vi "Test_WriteValue_InvalidRefnum_Error.vi"(8 "error in (no error)":errorcluster, 11 "TestCase in":refnum<class "TestStreamToDiskTransport.lvclass">) -> (0 "error out":errorcluster, 3 "TestCase out":refnum<class "TestStreamToDiskTransport.lvclass">)   [LabVIEW 2017, in "TestStreamToDiskTransport.lvclass"]
uses:
  TestStreamToDiskTransport.lvclass
  TestStreamToDiskTransport.lvclass/TestStreamToDiskTransport.ctl
  Source/Concrete/StreamToDiskTransport/StreamToDiskTransport.lvclass/StreamToDiskTransport.ctl
  <vilib>/Utility/error.llb/Clear Errors.vi
  Source/Concrete/StreamToDiskTransport/StreamToDiskTransport.lvclass
  C:/Git/composed-transport/Source/ITransport/ITransport.lvclass
  Source/ITransport/ITransport.lvclass
panel:
  out "Return Error":errorcluster
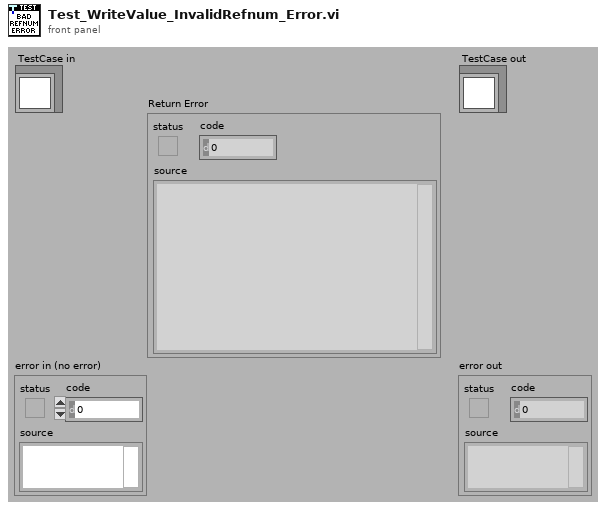
[diagram p1: front panel]
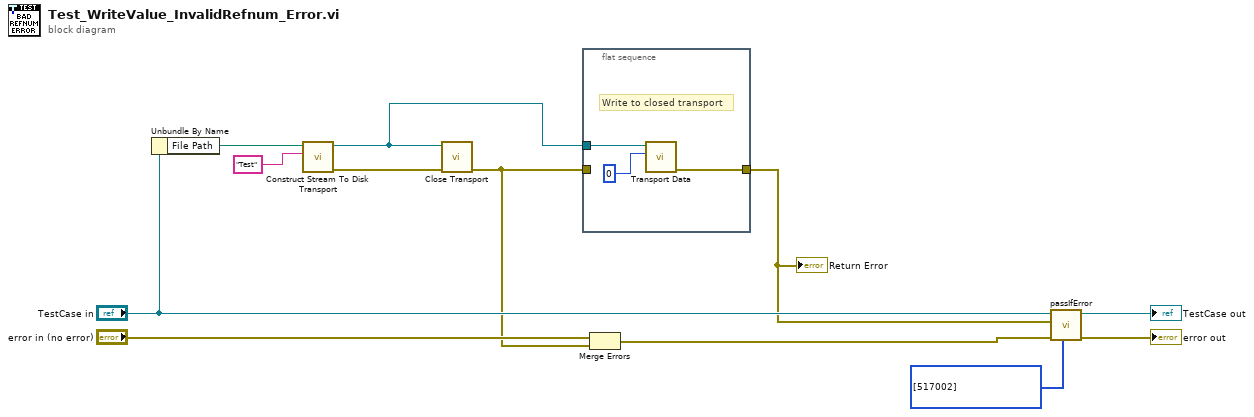
[diagram p0: block diagram]
diagram:
  n1 = Unbundle By Name("TestCase in") -> ("File Path"=w7:path)
  n2 = call "Construct Stream To Disk Transport.vi"("Channel Name"="Test" ("Section Name"), "File Path"=w7) -> ("error out"=w3:errorcluster, "StreamToDiskTransport"=w2:refnum<class "StreamToDiskTransport.lvclass">)  [unwired: 8 in]
  n3 = call-dynamic "Close Transport.vi"("error in (no error)"=w3, "StreamToDiskTransport"=w2) -> ("error out"=w1:errorcluster)  [unwired: 9 in]
  n4 = flat-sequence {
    tunnel: [w15] -> w5
    tunnel: w2 -> [w14]
    tunnel: w1 -> [_]
    frame #0 {
      # "Write to closed transport"
      n5 = call "Transport Data.vi"("Value"=0, "ITransport in"=w14) -> ("error out"=w15:errorcluster)  [unwired: 8 in, 1 out]
    }
  }
  n6 = Merge Errors("error in (no error)", w1) -> (w9:errorcluster)
  n7 = call-dynamic "passIfError.vi"("passing error codes (default = any error code)"=i32[] [517002], "error in (no error)"=w9, "error"=w5, "TestCase in"="TestCase in") -> ("error out"=→"error out":errorcluster, "TestCase out"=→"TestCase out":refnum<class "TestStreamToDiskTransport.lvclass">)  [unwired: 6 in]
  "Return Error" <- w5
